vi "create.ReduceSizeShort.vi"(8 "error in (no error)":errorcluster, 11 "ReduceSizeShort.Parameters":T1={"Time Offset"=447000, "Order Id"="ORID0001", "Canceled Quantity"=20000}) -> (0 "error out":errorcluster, 2 "Bytes.out":u8[](array[numeric]) format="%.0x", 3 "MessageBase out":refnum<class "ReduceSizeShort.lvclass">)   [LabVIEW 2020]
uses:
  ReduceSize/ReduceSizeShort.Parameters.ctl
  ReduceSize/ReduceSizeShort.lvclass
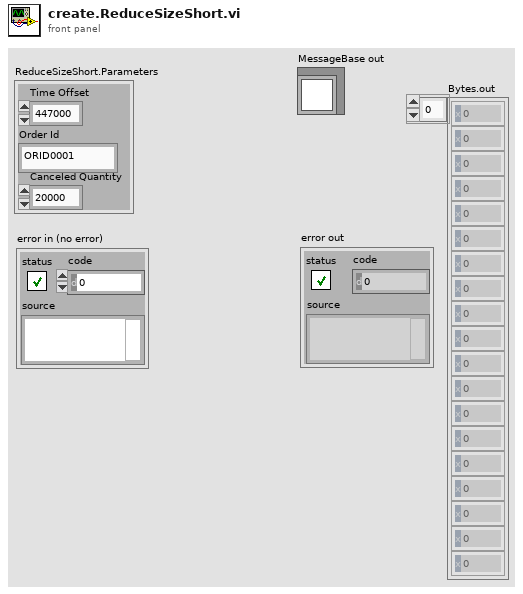
[diagram p1: front panel]
types:
  T1 = typedef "ReduceSizeShort.lvclass/ReduceSizeShort.Parameters.ctl" = cluster{"Time Offset":u32, "Order Id":string, "Canceled Quantity":u16}
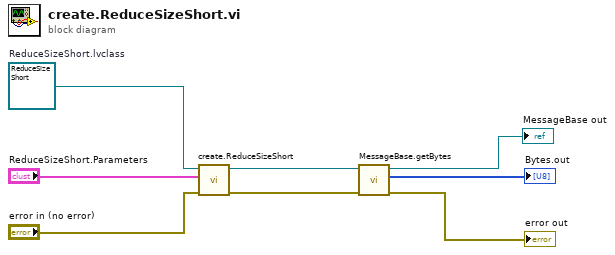
[diagram p0: block diagram]
diagram:
  w2 = refnum<class "ReduceSizeShort.lvclass"> refnum  # ReduceSizeShort.lvclass
  n1 = call-dynamic "create.ReduceSizeShort.vi"("error in"="error in (no error)", "ReduceSizeShort.Parameters"="ReduceSizeShort.Parameters", "ReduceSizeShort in"=w2) -> ("error out"=w6:errorcluster, "ReduceSizeShort out"=w7:refnum<class "ReduceSizeShort.lvclass">)  [unwired: 7 in]
  n2 = call-dynamic "MessageBase.getBytes.vi"("error in (no error)"=w6, "MessageBase in"=w7) -> ("error out"=→"error out":errorcluster, "Bytes.out"=→"Bytes.out":u8[], "MessageBase out"=→"MessageBase out":refnum<class "ReduceSizeShort.lvclass">)  [unwired: 7 in]
